vi "UT - Create HDF File.vi"(8 "error in (no error)":errorcluster, 10 "Dims 2":u64[](array[numeric]), 11 "Dims":u64[](array[numeric])) -> (0 "error out":errorcluster, 2 "Object Types":T1[](array[typedef]) items=["H5G_UNKNOWN"=-1, "H5G_GROUP"=0, "H5G_DATASET"=1, "H5G_TYPE"=2, "H5G_LINK"=3, "H5G_UDLINK"=4], 3 "Object Names":string[](array[string]))   [LabVIEW 2019]
uses:
  <vilib>/UPVI/lvhdf5/group.llb/H5G_obj_t.ctl
  <vilib>/UPVI/lvhdf5/file.llb/LVH5F Operation.ctl
  HDF5 Tools.lvlib
panel:
  out "Numeric":i32
  out "Unique Temporary File Path":path
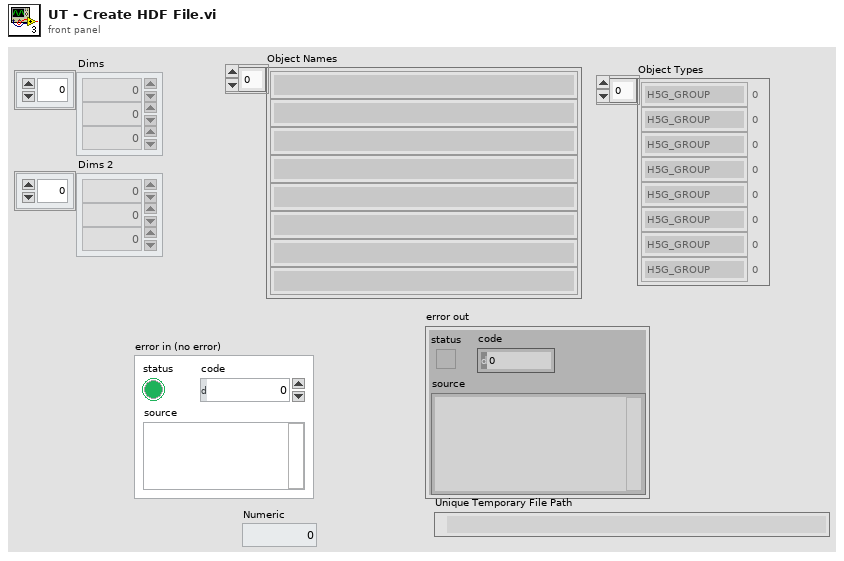
[diagram p1: front panel]
types:
  T1 = typedef "H5G_obj_t.ctl" = i32
  T2 = typedef "LVH5F Operation.ctl" = enum16{"open", "open or create", "create or replace", "create or replace (with confirmation)", "create", "open (read only)"}
  T3 = cluster{"My Numeric":dbl, "My Array":dbl[][], "My Inner Cluster":cluster{"My Numeric in Cluster":dbl}}
  T4 = typedef "HDF5 Ref.ctl" = refnum<k1>
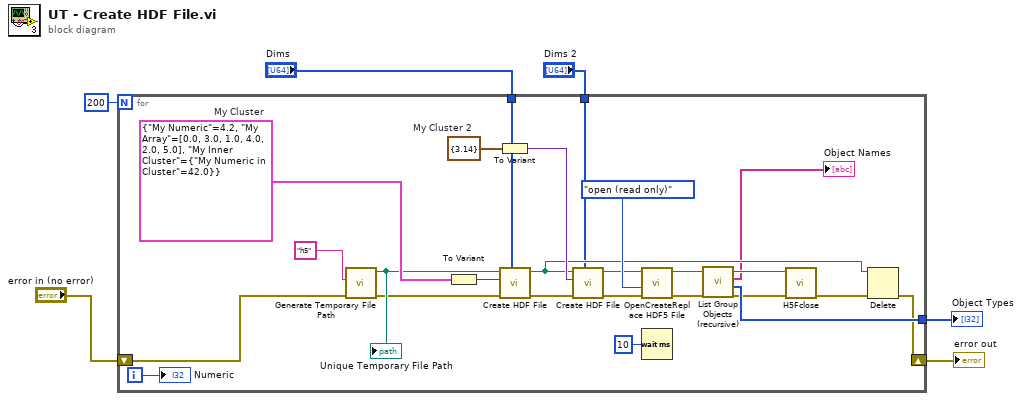
[diagram p0: block diagram]
diagram:
  n1 = for {
    N: 200 -> [_]
    tunnel: [w30] -> w6
    tunnel: "Dims" -> [w11]
    tunnel: "Dims 2" -> [w10]
    shift-right: [w23] -> w5
    shift-left: "error in (no error)" -> [w20]
    i -> [w8]
    w15 = cluster{"My Numeric":dbl} {"My Numeric"=3.14}  # My Cluster 2
    w25 = T3 {"My Numeric"=4.2, "My Array"=[[0.0, 3.0], [1.0, 4.0], [2.0, 5.0]], "My Inner Cluster"={"My Numeric in Cluster"=42.0}}  # My Cluster
    n2 = call <vilib>:"Generate Temporary File Path.vi"("error in (no error)"=w20, "Temporary File Extension (tmp)"="h5") -> ("error out"=w19:errorcluster, "Unique Temporary File Path"=w21:path)  [unwired: 8 in]
    "Unique Temporary File Path" <- w21
    n3 = To Variant(anything=w25) -> (Variant=w24:variant)
    n4 = To Variant(anything=w15) -> (Variant=w14:variant)
    n5 = call "Create HDF File.vi"("Dims"=w11, "error in (no error)"=w19, "variant"=w24, "path"=w21) -> ("error out"=w17:errorcluster, "path out"=w13:path)  [unwired: 5 in, 1 out]
    n6 = call "Create HDF File.vi"("Dims"=w10, "error in (no error)"=w17, "variant"=w14, "path"=w13) -> ("error out"=w16:errorcluster, "path out"=w12:path)  [unwired: 5 in, 1 out]
    n7 = call <vilib>:"OpenCreateReplace HDF5 File.vi"("error in (no error)"=w16, "function (open or create)"=LVH5F_Operation."open (read only)", "path"=w12) -> ("error out"=w26:errorcluster, "HDF5 Ref out"=w27:T4)  [unwired: 5 in]
    n8 = Wait (ms)(milliseconds to wait=u32 10) -> ()  [unwired: 1 out]
    n9 = call <vilib>:"List Group Objects (recursive).vi"("error in (no error)"=w26, "HDF5 Loc Ref"=w27) -> ("error out"=w29:errorcluster, "Object Types"=w30:T1[], "Object Names"=→"Object Names":string[], "HDF5 Loc Ref out"=w28:T4)  [unwired: 4 in]
    n10 = call <vilib>:"H5Fclose.vi"("error in (no error)"=w29, "HDF5 Ref"=w28) -> ("error out"=w31:errorcluster)  [unwired: 7 in]
    n11 = Delete(path (use dialog)=w13, error in=w31) -> (error out=w23:errorcluster)  [unwired: 3 in, 2 out]
    "Numeric" <- w8
  }
  "Object Types" <- w6
  "error out" <- w5
